vi "ztrsv - Solve Linear Eqs (Triangle, single) (CDB).vi"(4 "diagonal":T1 items=["Non-unit", "Unit"], 7 "operation A":T2 items=["Direct", "Conjugated & Transposed", "Transposed"], 8 "matrix A type":T3=3 items=["Lower Triangular"=2, "Upper Triangular"=3], 10 "x":cdb[](array[numeric]), 11 "A":T4) -> (0 "error":i32, 3 "ztrsv":cdb[](array[numeric]))   [LabVIEW 2018, in "NI_AALBLAS.lvlib"]
doc: "Solves the linear equation op(<B>A</B>)*<B>trsv</B> = <B>x</B> for <B>trsv</B>."
uses:
  NI_AALBLAS.lvlib
  ComplexMatrix.ctl
  LV_UpLo.ctl
  LV_Transpose.ctl
  LV_Diag.ctl
  Order.ctl
  Fucntion.ctl
  BLAS2 Utility(CDB).vi
  NI_Matrix.lvlib
panel:
  # "-1"
  # "ztrsv=op(A)  *x"
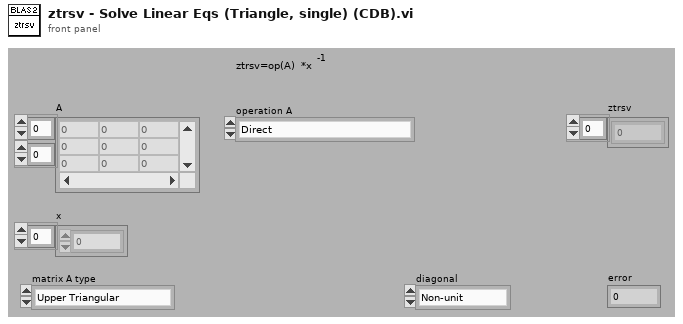
[diagram p1: front panel]
types:
  T1 = typedef "NI_AALBLAS.lvlib/LV_Diag.ctl" = i32
  T2 = typedef "NI_AALBLAS.lvlib/LV_Transpose.ctl" = i32
  T3 = typedef "NI_AALBLAS.lvlib/LV_UpLo.ctl" = i32
  T4 = typedef "NI_Matrix.lvlib/ComplexMatrix.ctl" = cdb[][]
  T5 = typedef "NI_AALBLAS.lvlib/Fucntion.ctl" = u16
  T6 = typedef "NI_AALBLAS.lvlib/Order.ctl" = i32
  T7 = typedef "NI_AALBLAS.lvlib/Diag.ctl" = i32
  T8 = typedef "NI_AALBLAS.lvlib/Operation_Transpose.ctl" = i32
  T9 = typedef "NI_AALBLAS.lvlib/UpLo.ctl" = i32
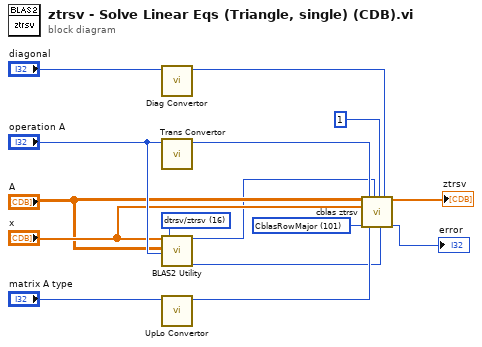
[diagram p0: block diagram]
diagram:
  w2 = T5 16 items=["ddot/zdotu/zdotc", "daxpy/zaxpy", "dnrm2/dznrm2", "dasum/dzasum", "dcopy/zcopy", "dswap/zswap", "drotm", "drot/zdrot", "idamax/izamax", "idamin/izamin", "dgemv/zgemv", "dsymv/zhemv", "dtrmv/ztrmv", "dsyr/zher", "dsyr2/zher2", "dger/zgeru/zgerc", "dtrsv/ztrsv", "dgemm/zgemm", "dsymm/zsymm/zhemm", "dtrmm/ztrmm", "dsyrk/zsyrk/zherk", "dsyr2k/zsyr2k/zher2k", "dtrsm/ztrsm"] ("function")
  w7 = T6 101 items=["CblasRowMajor"=101, "CblasColMajor"=102] ("order")
  n1 = call "Diag Convertor.vi"("diagonal"="diagonal") -> ("diag"=w10:T7)  [unwired: 10 out]
  n2 = call "Trans Convertor.vi"("operation"="operation A") -> ("trans"=w12:T8)  [unwired: 10 out]
  n3 = call-poly "BLAS2 Utility.vi"("x"="x", "A"="A", "operation A"="operation A", "function"=w2) -> ("lda"=w4:i32, "n"=w3:i32)  [unwired: 1 in, 13 out]
  n4 = call "UpLo Convertor.vi"("triangle matrix type"="matrix A type") -> ("uplo"=w11:T9)  [unwired: 10 out]
  n5 = call "cblas ztrsv.vi"("A"="A", "x"="x", "order"=w7, "transA"=w12, "uplo"=w11, "lda"=w4, "incx"=1 ("incX"), "n"=w3, "diag"=w10) -> ("ztrsv"=→"ztrsv":cdb[], "error"=→"error":i32)  [unwired: 9 out]
